vi "Prompt User for Path.vi"(8 "error in (no error)":errorcluster, 11 "ListBox in":refnum<vi>) -> (0 "error out":errorcluster, 3 "ListBox out":refnum<vi>)   [LabVIEW 2013, in "Example Configuration Dialog.lvlib" / "Example Configuration Dialog.lvclass"]
uses:
  Example Configuration Dialog.lvclass
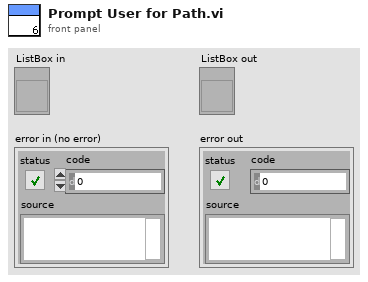
[diagram p1: front panel]
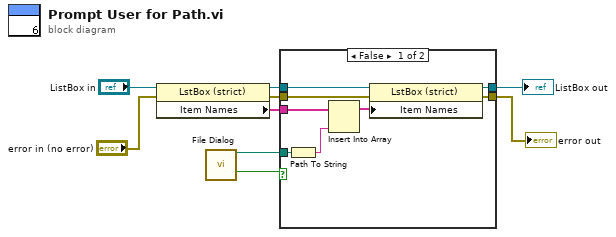
[diagram p0: block diagram]
diagram:
  n1 = property on="Property Node" class="LstBox (strict)"(reference="ListBox in", error in="error in (no error)") -> (reference out=w4:refnum<vi>, error out=w1:errorcluster, "Item Names"=w5:string[])
  n2 = call "File Dialog"() -> ("selected path"=w6:path, "cancelled"=w7:bool)  [unwired: 12 in, 2 out]
  n3 = case shown="False" w7 {
    tunnel: [w17 w19] -> w2
    tunnel: w4 -> [w16 w19]
    tunnel: w5 -> [w15 _]
    tunnel: w6 -> [w12 _]
    tunnel: [w11 w18] -> w9
    tunnel: w1 -> [w10 w18]
    frame False {
      n4 = Path To String(path=w12) -> (string=w13:string)
      n5 = Insert Into Array(array=w15, new element=w13) -> (w14:string[])  [unwired: 1 in]
      n6 = property on="Property Node" class="LstBox (strict)"(reference=w16, error in=w10, "Item Names"=w14) -> (reference out=w17:refnum<vi>, error out=w11:errorcluster)
    }
    frame True {
    }
  }
  "error out" <- w9
  "ListBox out" <- w2
